vi "Average Temperature.vi"() -> ()   [LabVIEW 2010]
doc: "This VI is the solution to an exercise in the LabVIEW Core I course.\n\nIt uses a For Loop and shift registers to average data. No hardware is necessary."
panel:
  out "Temperature History":dbl(graph)
  in  "Power":bool=TRUE
  # "ON\n\nOFF"
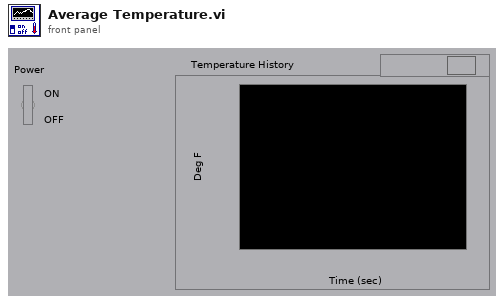
[diagram p1: front panel]
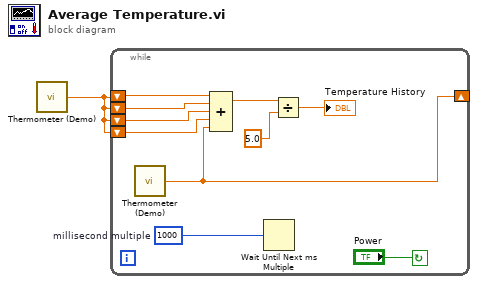
[diagram p0: block diagram]
diagram:
  n1 = call "Thermometer (Demo).vi"() -> ("Temperature"=w1:dbl)  [unwired: 1 in]
  n2 = while {
    shift-right: [w4] -> _
    shift-left: w1 -> [w9]
    shift-left: w1 -> [w8]
    shift-left: w1 -> [w3]
    shift-left: w1 -> [w2]
    stop <- "Power" continue-if-true
    w10 = u32 1000  # millisecond multiple
    n3 = call "Thermometer (Demo).vi"() -> ("Temperature"=w4:dbl)  [unwired: 1 in]
    n4 = Compound Arithmetic op=ADD(w9, w8, w3, w2, w4) -> (w7:dbl)
    n5 = Wait Until Next ms Multiple(millisecond multiple=w10) -> ()  [unwired: 1 out]
    n6 = Divide(x=w7, y=5.0) -> (x/y=→"Temperature History":dbl)
  }
